vi "LightState (SubVI).vi"(4 "Red in":refnum<vi>, 5 "Boolean":bool, 6 "White in":refnum<vi>, 7 "Button number(1-5)":dbl, 9 "Blue in":refnum<vi>, 10 "Yellow in":refnum<vi>, 11 "Boolean in":refnum<vi>) -> ()   [LabVIEW 2014]
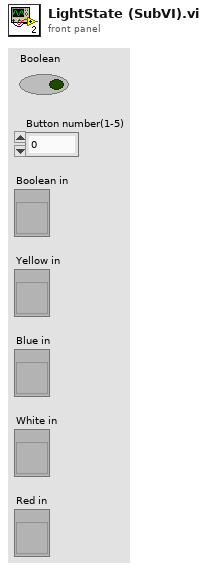
[diagram p1: front panel]
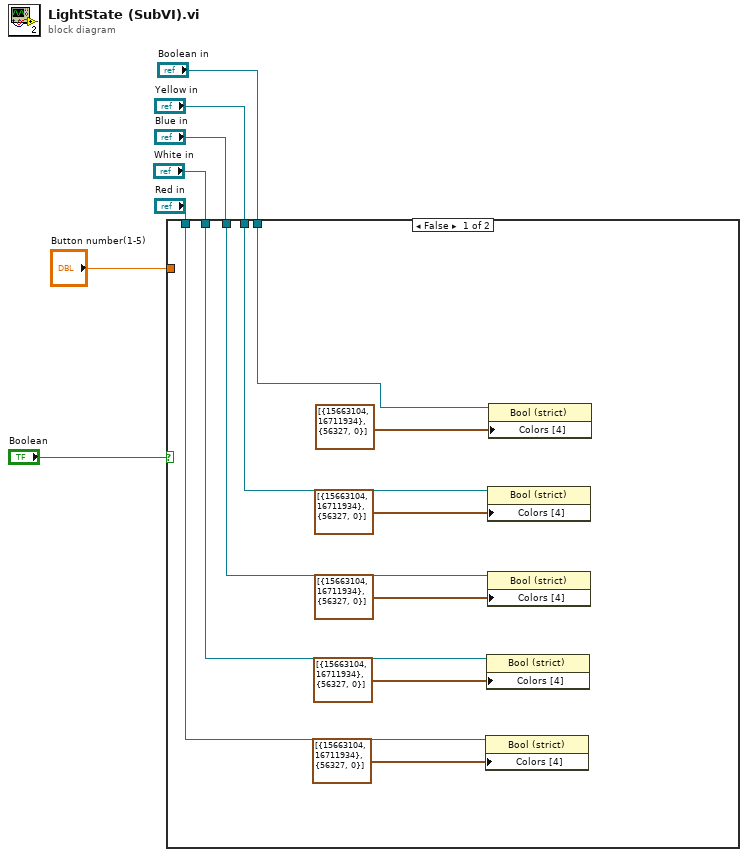
[diagram p0: block diagram]
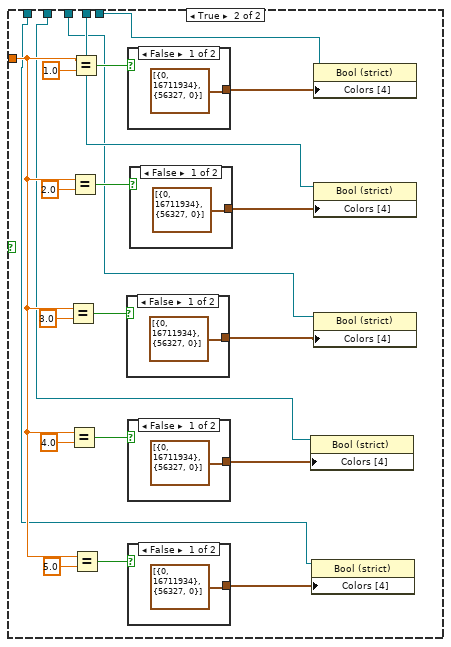
[diagram p2: hidden frame]
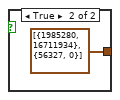
[diagram p3: hidden frame]
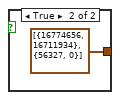
[diagram p4: hidden frame]
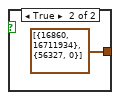
[diagram p5: hidden frame]
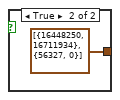
[diagram p6: hidden frame]
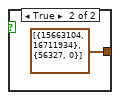
[diagram p7: hidden frame]
diagram:
  n1 = case shown="False" "Boolean" {
    tunnel: "Button number(1-5)" -> [_ w23]
    tunnel: "Boolean in" -> [w12 w22]
    tunnel: "Yellow in" -> [w11 w21]
    tunnel: "Blue in" -> [w10 w20]
    tunnel: "White in" -> [w9 w19]
    tunnel: "Red in" -> [w8 w18]
    frame False {
      n2 = property on="Property Node" class="Bool (strict)"(reference=w8, "Colors [4]"=cluster{u32, u32}[] [{15663104, 16711934}, {56327, 0}]) -> ()  [unwired: 1 in, 2 out]
      n3 = property on="Property Node" class="Bool (strict)"(reference=w9, "Colors [4]"=cluster{u32, u32}[] [{15663104, 16711934}, {56327, 0}]) -> ()  [unwired: 1 in, 2 out]
      n4 = property on="Property Node" class="Bool (strict)"(reference=w11, "Colors [4]"=cluster{u32, u32}[] [{15663104, 16711934}, {56327, 0}]) -> ()  [unwired: 1 in, 2 out]
      n5 = property on="Property Node" class="Bool (strict)"(reference=w10, "Colors [4]"=cluster{u32, u32}[] [{15663104, 16711934}, {56327, 0}]) -> ()  [unwired: 1 in, 2 out]
      n6 = property on="Property Node" class="Bool (strict)"(reference=w12, "Colors [4]"=cluster{u32, u32}[] [{15663104, 16711934}, {56327, 0}]) -> ()  [unwired: 1 in, 2 out]
    }
    frame True {
      n7 = Equal?(x=w23, y=3.0) -> (x = y?=w30:bool)
      n8 = Equal?(x=w23, y=4.0) -> (x = y?=w31:bool)
      n9 = Equal?(x=w23, y=2.0) -> (x = y?=w29:bool)
      n10 = Equal?(x=w23, y=1.0) -> (x = y?=w33:bool)
      n11 = Equal?(x=w23, y=5.0) -> (x = y?=w32:bool)
      n12 = case shown="False" w30 {
        tunnel: [cluster{u32, u32}[] [{0, 16711934}, {56327, 0}] cluster{u32, u32}[] [{16860, 16711934}, {56327, 0}]] -> w36
        frame False {
        }
        frame True {
        }
      }
      n13 = case shown="False" w33 {
        tunnel: [cluster{u32, u32}[] [{0, 16711934}, {56327, 0}] cluster{u32, u32}[] [{1985280, 16711934}, {56327, 0}]] -> w34
        frame False {
        }
        frame True {
        }
      }
      n14 = case shown="False" w31 {
        tunnel: [cluster{u32, u32}[] [{0, 16711934}, {56327, 0}] cluster{u32, u32}[] [{16448250, 16711934}, {56327, 0}]] -> w37
        frame False {
        }
        frame True {
        }
      }
      n15 = case shown="False" w32 {
        tunnel: [cluster{u32, u32}[] [{0, 16711934}, {56327, 0}] cluster{u32, u32}[] [{15663104, 16711934}, {56327, 0}]] -> w38
        frame False {
        }
        frame True {
        }
      }
      n16 = case shown="False" w29 {
        tunnel: [cluster{u32, u32}[] [{0, 16711934}, {56327, 0}] cluster{u32, u32}[] [{16774656, 16711934}, {56327, 0}]] -> w35
        frame False {
        }
        frame True {
        }
      }
      n17 = property on="Property Node" class="Bool (strict)"(reference=w19, "Colors [4]"=w37) -> ()  [unwired: 1 in, 2 out]
      n18 = property on="Property Node" class="Bool (strict)"(reference=w18, "Colors [4]"=w38) -> ()  [unwired: 1 in, 2 out]
      n19 = property on="Property Node" class="Bool (strict)"(reference=w22, "Colors [4]"=w34) -> ()  [unwired: 1 in, 2 out]
      n20 = property on="Property Node" class="Bool (strict)"(reference=w21, "Colors [4]"=w35) -> ()  [unwired: 1 in, 2 out]
      n21 = property on="Property Node" class="Bool (strict)"(reference=w20, "Colors [4]"=w36) -> ()  [unwired: 1 in, 2 out]
    }
  }
